vi "params.From JSON String.vi"(8 "error in (no error)":errorcluster, 10 "JSON String":string, 11 "params in":refnum<class "params.lvclass">) -> (0 "error out":errorcluster, 3 "params in":refnum<class "params.lvclass">)   [LabVIEW 2016, in "params.lvclass"]
uses:
  params.lvclass
  <vilib>/NI/JSON Support for LabVIEW/JSON Value/JSON Value.lvclass
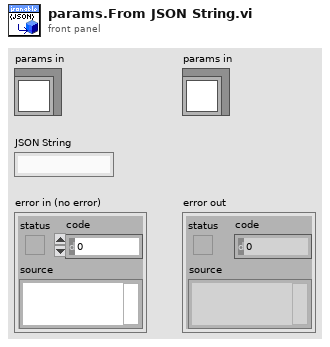
[diagram p1: front panel]
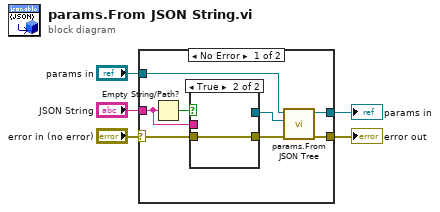
[diagram p0: block diagram]
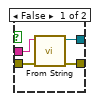
[diagram p2: hidden frame]
diagram:
  n1 = case shown="No Error" "error in (no error)" {
    selector: "error in (no error)" -> [w10 w20]
    tunnel: [w11 w20] -> w4
    tunnel: [w12 w19] -> w2
    tunnel: "params in" -> [w13 w19]
    tunnel: "JSON String" -> [w8 _]
    frame No Error {
      n2 = Empty String/Path?(string/path=w8) -> (empty?=w7:bool)
      n3 = case shown="True" w7 {
        tunnel: w8 -> [w17 _]
        tunnel: [w16 _] -> w6
        tunnel: w10 -> [w14 w18]
        tunnel: [w15 w18] -> w9
        frame False {
          n4 = call <vilib>:"From String.vi"("error in (no error)"=w14, "JSON String"=w17) -> ("error out"=w15:errorcluster, "JSON Value out"=w16:refnum<class "JSON Value.lvclass">)  [unwired: 8 in]
        }
        frame True {
        }
      }
      n5 = call "params.From JSON Tree.vi"("error in (no error)"=w9, "JSON Value in"=w6, "params in"=w13) -> ("error out"=w11:errorcluster, "params in"=w12:refnum<class "params.lvclass">)  [unwired: 7 in]
    }
    frame Error {
    }
  }
  "error out" <- w4
  "params in" <- w2
